vi "OPO_TCP_Client.vi"(8 "error in (no error)":errorcluster, 11 "port":u16=6000) -> (0 "error out":errorcluster)   [LabVIEW 2020]
panel:
  out "value read":dbl
  in  "stop":bool
  out "bytes written":i32
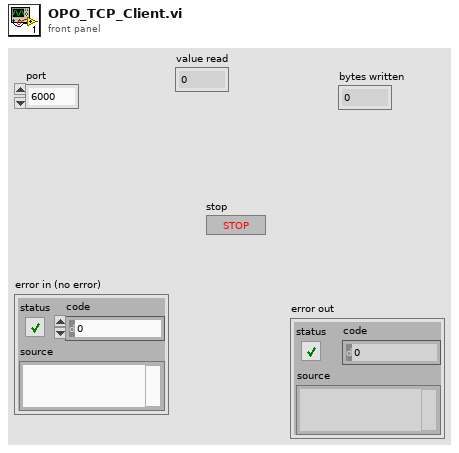
[diagram p1: front panel]
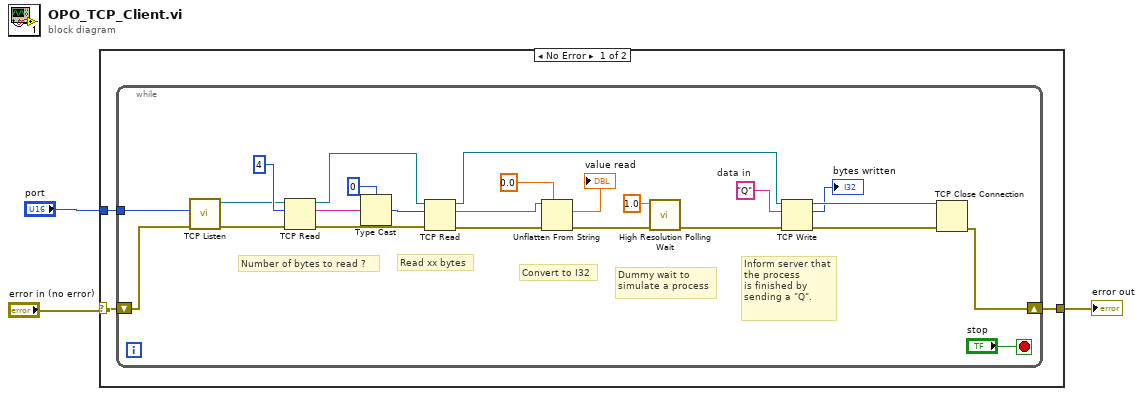
[diagram p0: block diagram]
diagram:
  n1 = case shown="No Error" "error in (no error)" {
    selector: "error in (no error)" -> [w5 w31]
    tunnel: [w4 w31] -> w2
    tunnel: "port" -> [w6 _]
    frame No Error {
      n2 = while {
        tunnel: w6 -> [w30]
        shift-right: [w28] -> w4
        shift-left: w5 -> [w29]
        stop <- "stop" stop-if-true
        w14 = "Q"  # data in
        # "Dummy wait to\nsimulate a process"
        # "Convert to I32"
        # "Inform server that the process\nis finished by sending a \"Q\"."
        # "Read xx bytes"
        # "Number of bytes to read ?"
        n3 = call <vilib>:"TCP Listen.vi"("error in (no error)"=w29, "port"=w30) -> ("error out"=w25:errorcluster, "connection ID"=w26:refnum<k5>)  [unwired: 5 in, 3 out]
        n4 = TCP Read(connection ID=w26, bytes to read=4, error in (no error)=w25) -> (connection ID out=w21:refnum<k5>, data out=w23:string, error out=w24:errorcluster)  [unwired: 2 in]
        n5 = Type Cast(type=0, x=w23) -> (*(type *) &x=w10:i32)
        n6 = TCP Read(connection ID=w21, bytes to read=w10, error in (no error)=w24) -> (connection ID out=w17:refnum<k5>, data out=w19:string, error out=w20:errorcluster)  [unwired: 2 in]
        n7 = Unflatten From String(type=0.0, binary string=w19, error in (no error)=w20) -> (value=→"value read":dbl, error out=w18:errorcluster)  [unwired: 2 in, 1 out]
        n8 = call <vilib>:"High Resolution Polling Wait.vi"("error in (no error)"=w18, "seconds to wait"=1.0) -> ("error out"=w12:errorcluster)  [unwired: 9 in]
        n9 = TCP Write(connection ID=w17, data in=w14, error in (no error)=w12) -> (connection ID out=w16:refnum<k5>, bytes written=→"bytes written":i32, error out=w15:errorcluster)  [unwired: 1 in]
        n10 = TCP Close Connection(connection ID=w16, error in (no error)=w15) -> (error out=w28:errorcluster)  [unwired: 1 in, 1 out]
      }
    }
    frame Error {
    }
  }
  "error out" <- w2
